vi "ReadSizeMat_1DArray-I64.vi"(8 "error in":errorcluster, 11 "Array in":i64[](array[numeric])) -> (0 "error out":errorcluster, 1 "Height":i32, 2 "Width":i32, 3 "Array out":i64[](array[numeric]), 4 "Channel":i32)   [LabVIEW 2020, in "OpenLvVision_OpenCv.lvlib"]
doc: "Read size of the datatype\nNo malleable to breake vi inlining!"
uses:
  OpenLvVision_OpenCv.lvlib
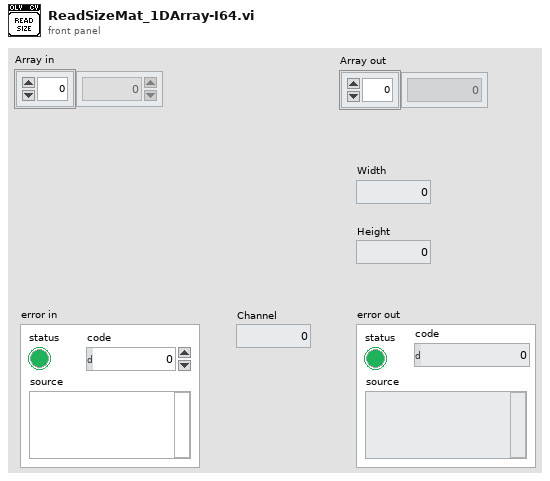
[diagram p1: front panel]
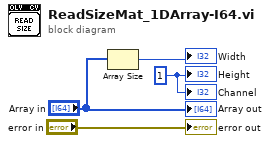
[diagram p0: block diagram]
diagram:
  w1 = 1
  n1 = Array Size(array="Array in") -> (size(s)=→"Width":i32)
  "error out" <- "error in"
  "Height" <- w1
  "Channel" <- w1
  "Array out" <- "Array in"
